vi "cuba.vi"() -> ()   [LabVIEW 2016, in "testing1.lvrbt"]
uses:
  testing1.lvrbt
  <vilib>/NXT/Subs/LVHSConnector.ctl
  <vilib>/NXT/LegoClasses/BrickReference/BrickReference.lvclass
  <vilib>/NXT/Hardware/Plugins/Tetrix 180 deg Servo/Tetrix180ServoAddress.ctl
  <vilib>/NXT/NXTIO Xnodes/NXTIONodeSubVIs/TETRIX IO Move Servos.vi
  <vilib>/NXT/Dual Mode Library/Waits/Wait_Num.vi
  <vilib>/NXT/NXTIO Xnodes/AddressXNode/NXTIOAddress.xnode
  <vilib>/NXT/NXTIO Xnodes/NXTIOXNode/NXTIO.xnode
panel:
  in  "stop":bool
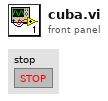
[diagram p1: front panel]
types:
  T1 = typedef "LVHSConnector.ctl" = refnum<class "BrickReference.lvclass">
  T2 = typedef "Tetrix180ServoAddress.ctl" = i32
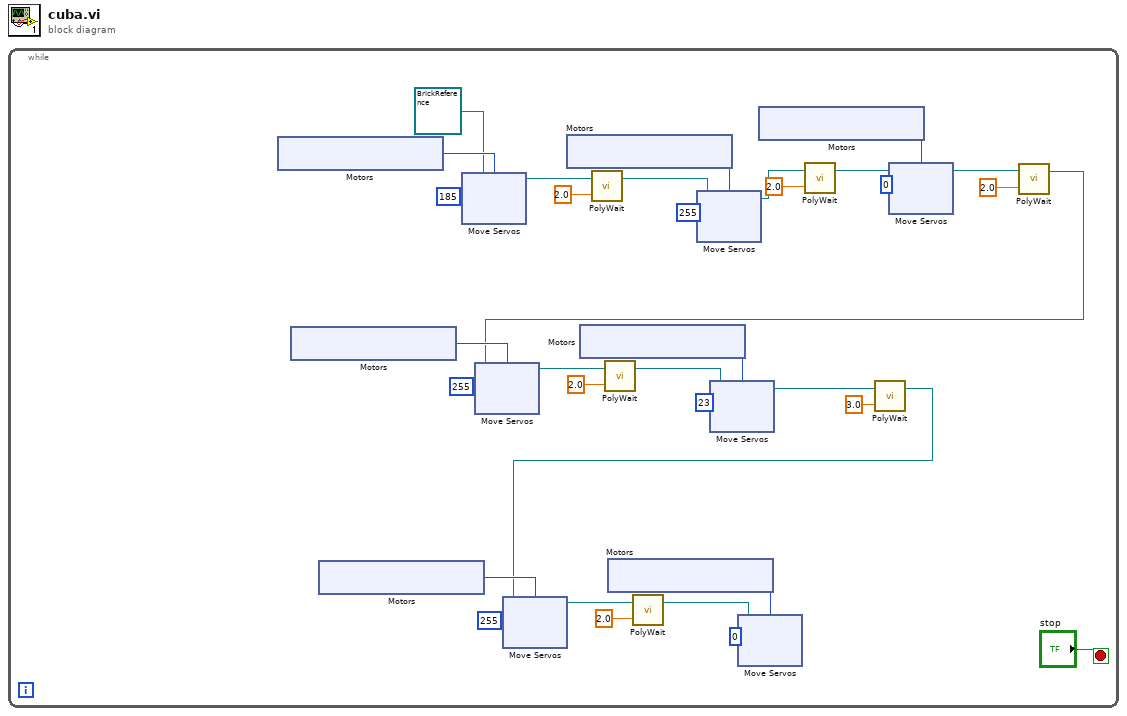
[diagram p0: block diagram]
diagram:
  n1 = while {
    stop <- "stop" stop-if-true
    n2 = xnode "Motors"() -> ("Motor"=w34:T2)
    n3 = xnode "Motors"() -> ("Motor"=w16:T2)
    n4 = xnode "Motors"() -> ("Motor"=w11:T2)
    n5 = xnode "Move Servos"("Position 1"=u8 185, "Motors"=w34, "NXT/EV3"=T1 refnum) -> ("NXT/EV3"=w32:T1)
    n6 = xnode "Motors"() -> ("Motor"=w30:T2)
    n7 = xnode "Motors"() -> ("Motor"=w20:T2)
    n8 = call-poly <vilib>:"PolyWait.vi"("Time (1 sec)"=sgl 2.0, "NXT/EV3"=w32) -> ("NXT/EV3"=w29:T1)  [unwired: 2 in]
    n9 = xnode "Motors"() -> ("Motor"=w7:T2)
    n10 = xnode "Move Servos"("Position 1"=u8 255, "Motors"=w30, "NXT/EV3"=w29) -> ("NXT/EV3"=w25:T1)
    n11 = xnode "Motors"() -> ("Motor"=w27:T2)
    n12 = call-poly <vilib>:"PolyWait.vi"("Time (1 sec)"=sgl 2.0, "NXT/EV3"=w25) -> ("NXT/EV3"=w23:T1)  [unwired: 2 in]
    n13 = xnode "Move Servos"("Position 1"=u8 0, "Motors"=w27, "NXT/EV3"=w23) -> ("NXT/EV3"=w14:T1)
    n14 = call-poly <vilib>:"PolyWait.vi"("Time (1 sec)"=sgl 2.0, "NXT/EV3"=w14) -> ("NXT/EV3"=w1:T1)  [unwired: 2 in]
    n15 = xnode "Move Servos"("Position 1"=u8 255, "Motors"=w16, "NXT/EV3"=w1) -> ("NXT/EV3"=w18:T1)
    n16 = call-poly <vilib>:"PolyWait.vi"("Time (1 sec)"=sgl 2.0, "NXT/EV3"=w18) -> ("NXT/EV3"=w21:T1)  [unwired: 2 in]
    n17 = xnode "Move Servos"("Position 1"=u8 23, "Motors"=w20, "NXT/EV3"=w21) -> ("NXT/EV3"=w13:T1)
    n18 = call-poly <vilib>:"PolyWait.vi"("Time (1 sec)"=sgl 3.0, "NXT/EV3"=w13) -> ("NXT/EV3"=w2:T1)  [unwired: 2 in]
    n19 = xnode "Move Servos"("Position 1"=u8 255, "Motors"=w11, "NXT/EV3"=w2) -> ("NXT/EV3"=w9:T1)
    n20 = call-poly <vilib>:"PolyWait.vi"("Time (1 sec)"=sgl 2.0, "NXT/EV3"=w9) -> ("NXT/EV3"=w6:T1)  [unwired: 2 in]
    n21 = xnode "Move Servos"("Position 1"=u8 0, "Motors"=w7, "NXT/EV3"=w6) -> ()  [unwired: 1 out]
  }
